vi "Query External Input Line Overrun Status.vi"(8 "error in (no error)":errorcluster, 11 "VISA resource name":refnum<visa-resource-name>) -> (0 "error out":errorcluster, 2 "Overrun Status":i32, 3 "VISA resource name out":refnum<visa-resource-name>)   [LabVIEW 2016, in "Keithley DMM7510.lvlib"]
doc: "This VI returns the External Trigger event detector overrun status."
uses:
  Keithley DMM7510.lvlib
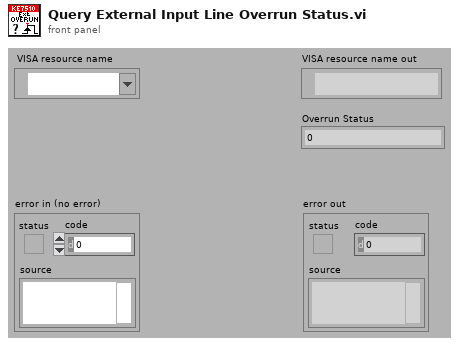
[diagram p1: front panel]
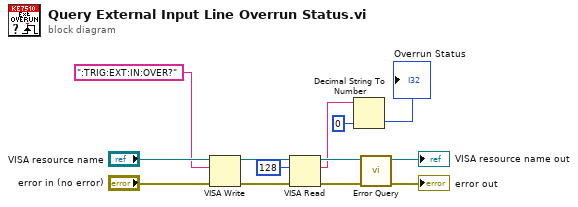
[diagram p0: block diagram]
diagram:
  n1 = VISA Write(VISA resource name="VISA resource name", write buffer=":TRIG:EXT:IN:OVER?" ("format string"), error in (no error)="error in (no error)") -> (VISA resource name out=w7:refnum<visa-resource-name>, error out=w9:errorcluster)  [unwired: 1 out]
  n2 = VISA Read(VISA resource name=w7, byte count=u32 128, error in (no error)=w9) -> (VISA resource name out=w6:refnum<visa-resource-name>, read buffer=w4:string, error out=w8:errorcluster)  [unwired: 1 out]
  n3 = Decimal String To Number(string=w4, default (0L)=0 ("default (0 I32)")) -> (number=→"Overrun Status":i32)  [unwired: 1 in, 1 out]
  n4 = call "Error Query.vi"("error in (no error)"=w8, "VISA resource name"=w6) -> ("error out"=→"error out":errorcluster, "VISA resource name out"=→"VISA resource name out":refnum<visa-resource-name>)  [unwired: 8 out]
